vi "ConvertToPolarVector.vi"(8 "error in (no error)":errorcluster, 11 "CartesianVector in":refnum<class "CartesianVector.lvclass">) -> (0 "error out":errorcluster, 3 "PolarVector.lvclass":refnum<class "PolarVector.lvclass">)   [LabVIEW 2011, in "CartesianVector.lvclass"]
doc: "Converts a CartesianVector object to a PolarVector object."
uses:
  CartesianVector.lvclass
  PolarVector/PolarVector.lvclass
  CartesianVector.lvclass/CartesianVector.ctl
  PolarVector/Initialize_DBL.vi
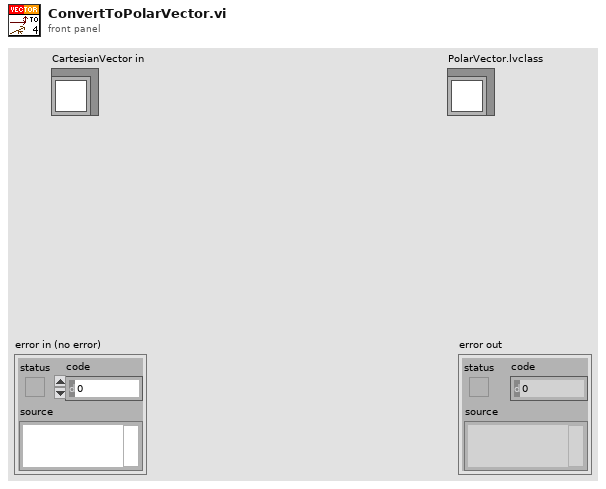
[diagram p1: front panel]
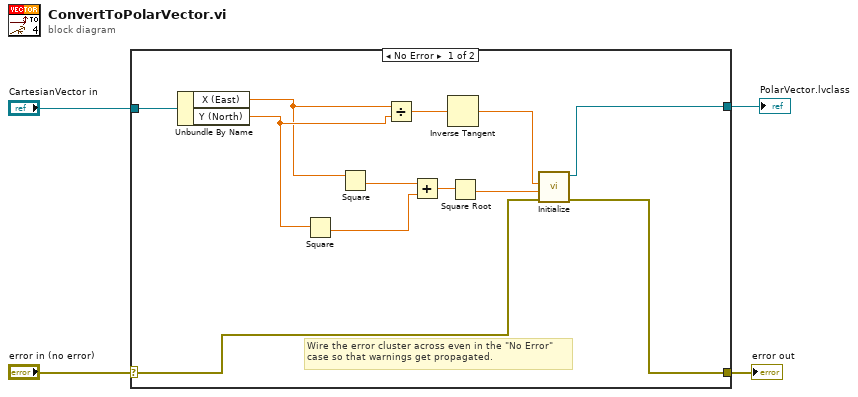
[diagram p0: block diagram]
diagram:
  n1 = case shown="No Error" "error in (no error)" {
    selector: "error in (no error)" -> [w6 w17]
    tunnel: [w5 w17] -> w3
    tunnel: "CartesianVector in" -> [w16 _]
    tunnel: [w9 _] -> w1
    frame No Error {
      # "Wire the error cluster across even in the \"No Error\"\ncase so that warnings get propagated."
      n2 = Unbundle By Name(w16) -> ("X (East)"=w11:dbl, "Y (North)"=w12:dbl)
      n3 = Square(x=w12) -> (x^2=w14:dbl)
      n4 = Square(x=w11) -> (x^2=w15:dbl)
      n5 = Divide(x=w11, y=w12) -> (x/y=w10:dbl)
      n6 = Add(x=w15, y=w14) -> (x+y=w13:dbl)
      n7 = Inverse Tangent(1:w10) -> (0:w8:dbl)
      n8 = Square Root(x=w13) -> (sqrt(x)=w7:dbl)
      n9 = call-poly "Initialize.vi"("error in (no error)"=w6, "Radius"=w7, "Angle (degrees)"=w8) -> ("error out"=w5:errorcluster, "PolarVector out"=w9:refnum<class "PolarVector.lvclass">)  [unwired: 7 in]
    }
    frame Error {
    }
  }
  "error out" <- w3
  "PolarVector.lvclass" <- w1
